vi "Generate SciScan specific XML params.vi"(8 "error in (no error)":errorcluster, 10 "DOM document IN":refnum<k20>, 11 "Non-Tree elements 2D array IN":string[][](array[string])) -> (0 "error out":errorcluster, 3 "Path-Value pairs Array":cluster{"XML Path":string, "XML Value":string}[](array[cluster]))   [LabVIEW 2012]
doc: "SciScan 1.2 160622"
uses:
  Custom Controls/file format type def.ctl
  Custom Controls/scan mode main settings tab.ctl
  GFG/GFGpathGet.vi
  GFG/GFG library.lvlib
  <resource>/objmgr/DOMUserDefRef.rc
  <vilib>/xml/NI_XML.lvlib
panel:
  out "node out":refnum<k20>
  in  "Channels 2 D Array IN":string[][](array[string])
  out "Array":string[](array[string])
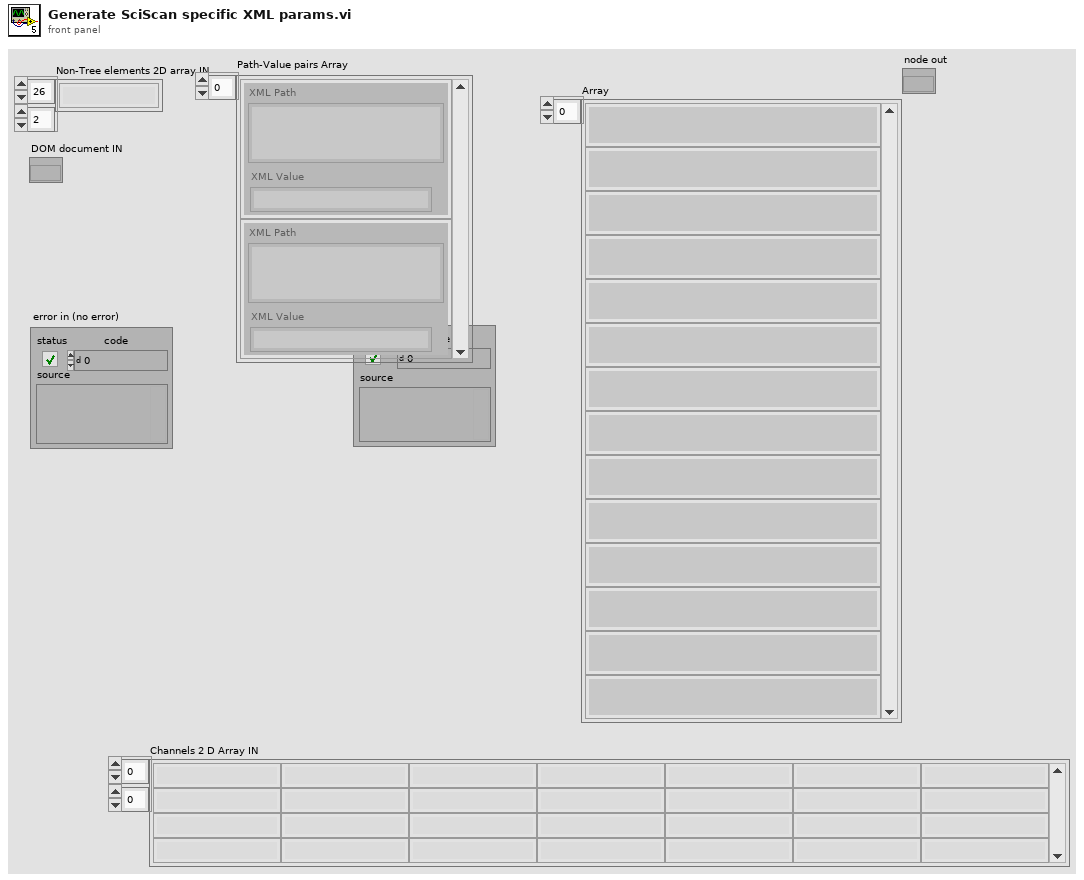
[diagram p1: front panel]
types:
  T1 = typedef "file format type def.ctl" = enum16{"16bit raw", "32bit raw", "16bit multi-tiff (interleave)", "16bit multi-tiff (separate)", "16bit multi-tiff (stacked)", "32bit multi-tiff (interleave)", "32bit multi-tiff (separate)", "32bit multi-tiff (stacked)", "16bit tiff series (interleave)", "16bit tiff series (separate)", "16bit tiff series (stacked)", "32bit tiff series (interleave)", "32bit tiff series (separate)", "32bit tiff series (stacked)"}
  T2 = typedef "scan mode main settings tab.ctl" = enum32{"2D frame", "2D line scan", "general settings", "Z Stack", "piezo"}
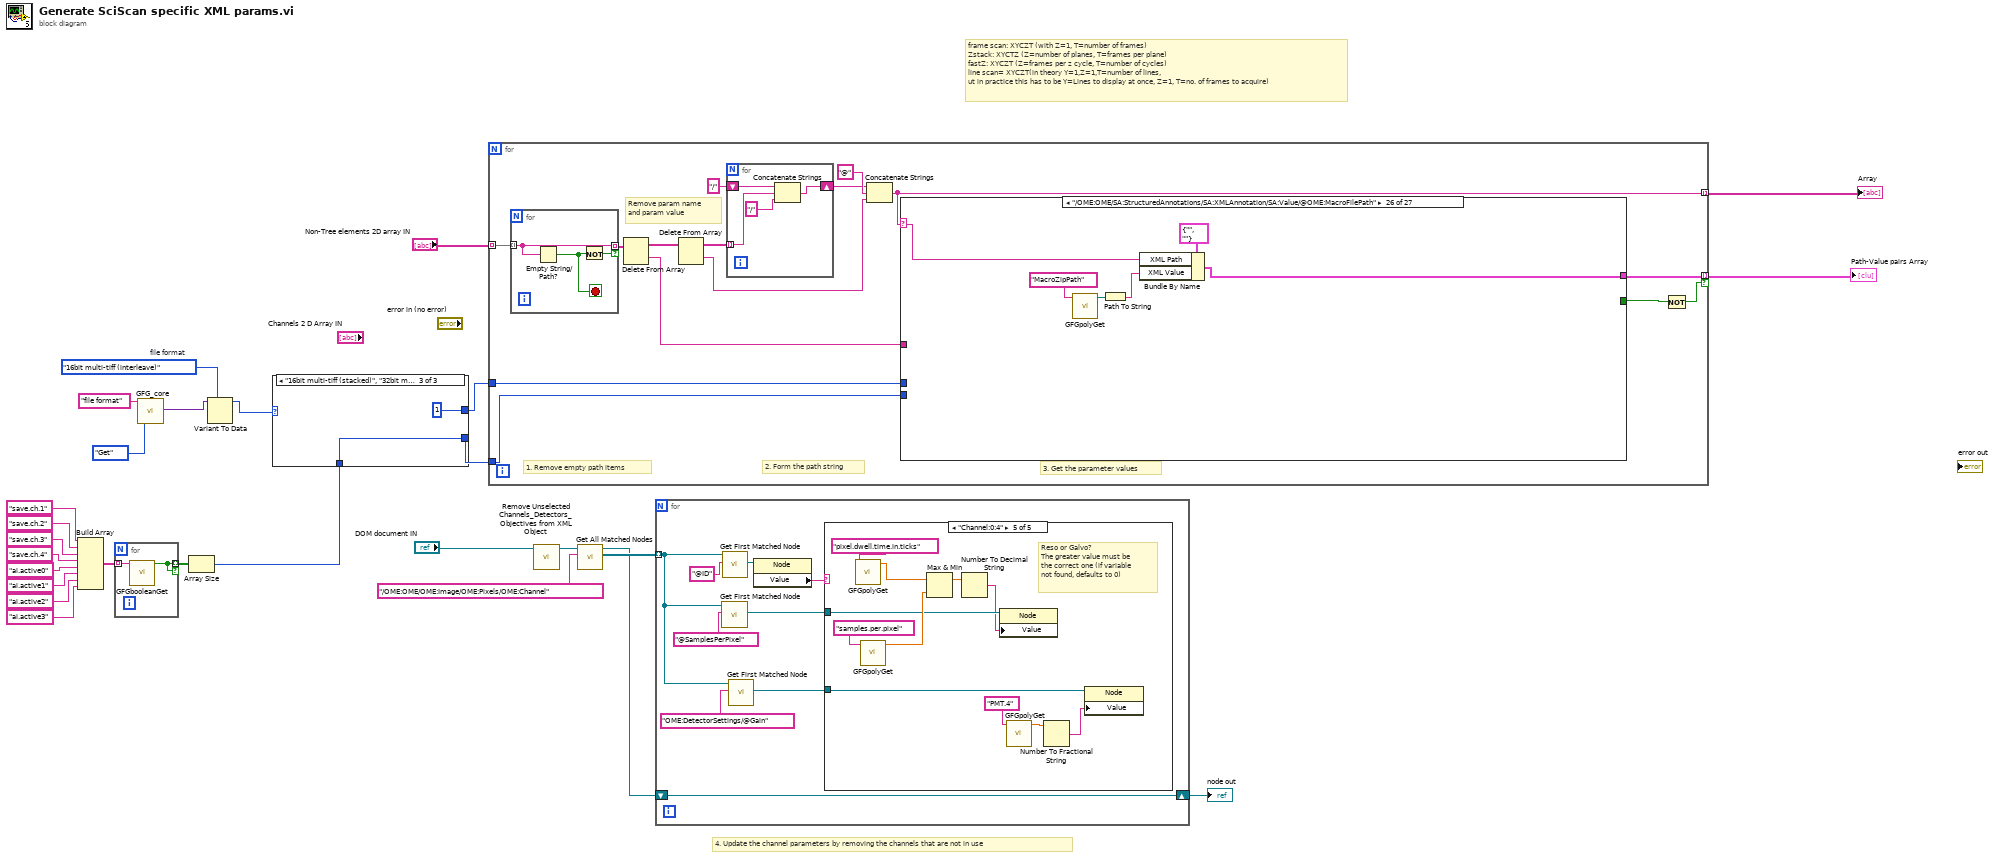
[diagram p0: block diagram]
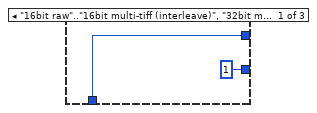
[diagram p2: hidden frame]
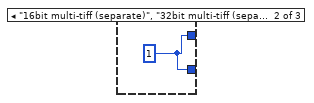
[diagram p3: hidden frame]
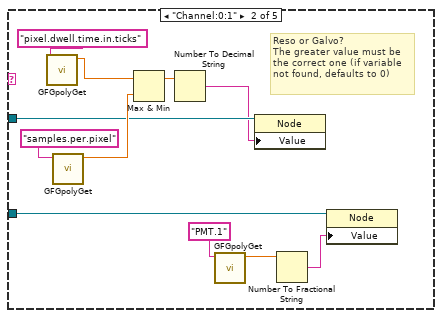
[diagram p5: hidden frame]
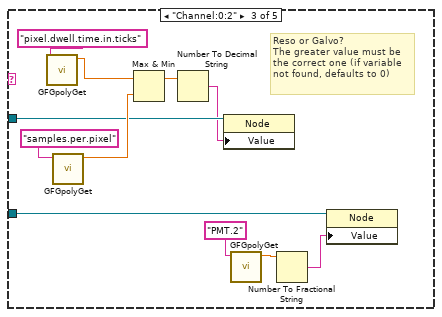
[diagram p6: hidden frame]
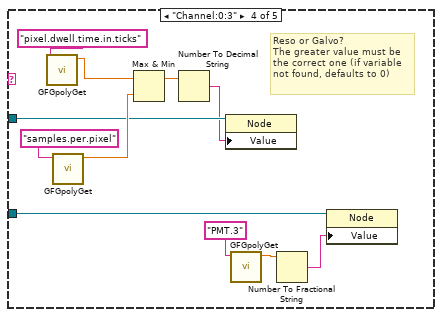
[diagram p7: hidden frame]
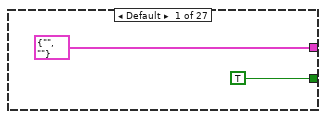
[diagram p8: hidden frame]
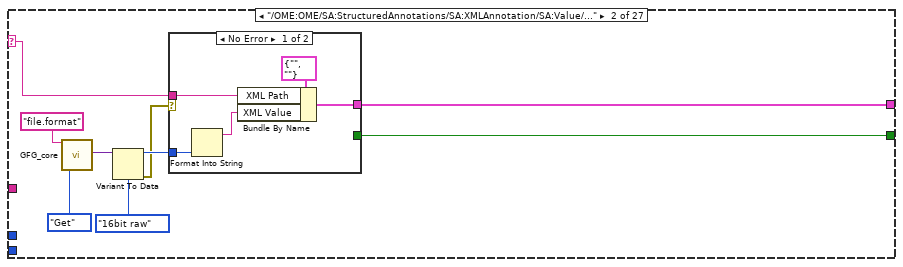
[diagram p9: hidden frame]
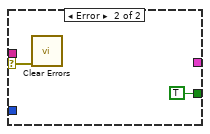
[diagram p10: hidden frame]
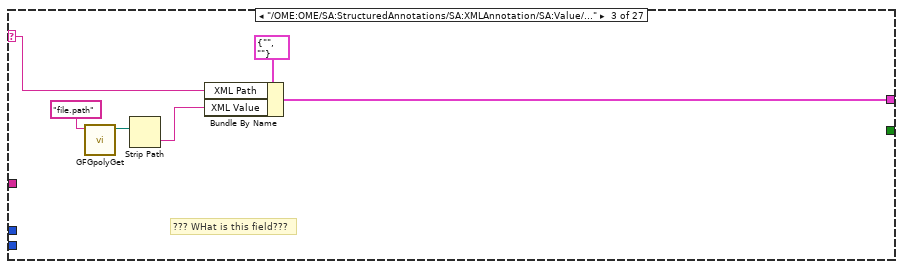
[diagram p11: hidden frame]
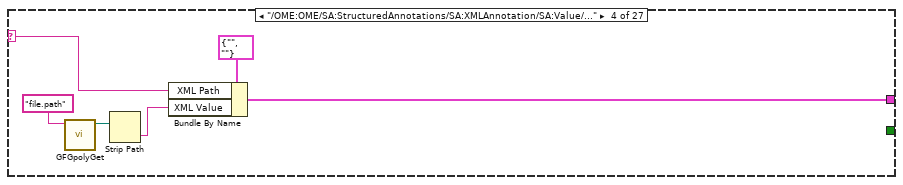
[diagram p12: hidden frame]
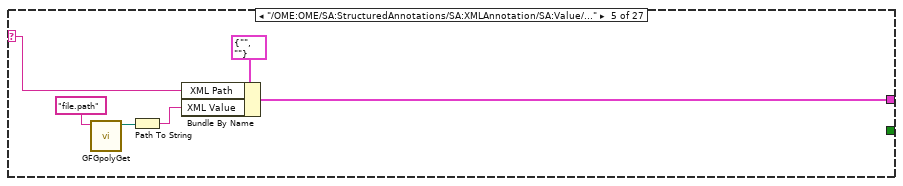
[diagram p13: hidden frame]
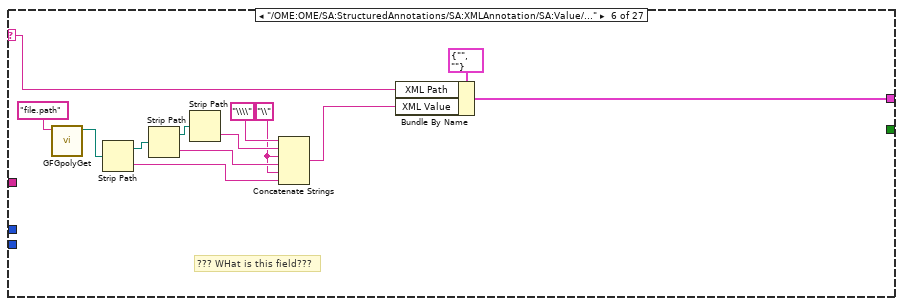
[diagram p14: hidden frame]
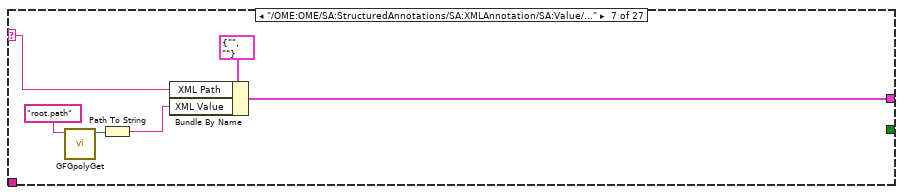
[diagram p15: hidden frame]
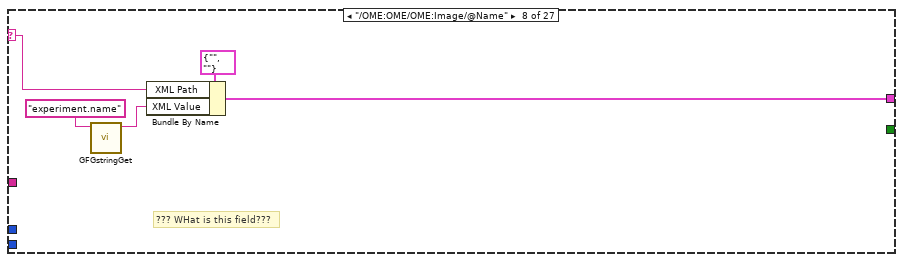
[diagram p16: hidden frame]
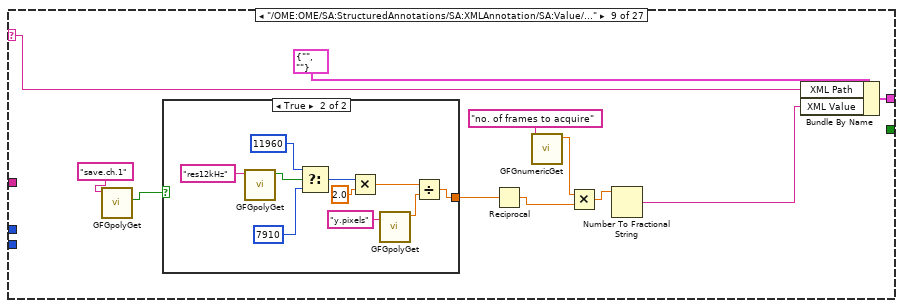
[diagram p17: hidden frame]
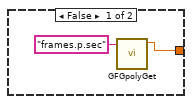
[diagram p18: hidden frame]
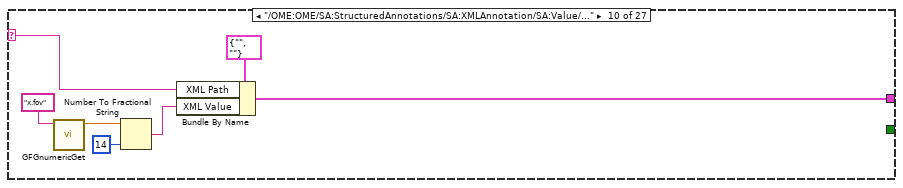
[diagram p19: hidden frame]
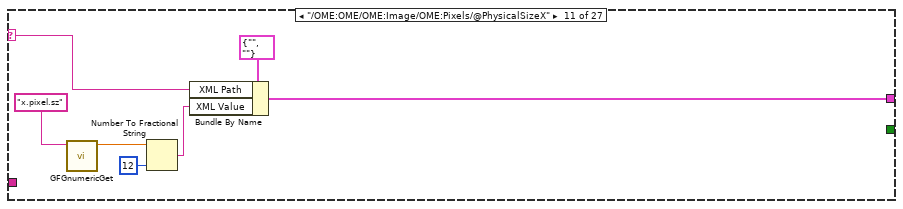
[diagram p20: hidden frame]
diagram:
  w16 = file_format_type_def."16bit multi-tiff (interleave)"  # file format
  # "frame scan: XYCZT (with Z=1, T=number of frames)\nZstack: XYCTZ (Z=number of planes, T=frames per plane)\nfastZ: XYCZT (Z=frames per z cycle, T=number of cycles)\nline scan= XYCZT(in theory Y=1,Z=1,T=number of lines, \nut in practice this has to be Y=Lines to display at once, Z=1, T=no. of frames to acquire)"
  # "4. Update the channel parameters by removing the channels that are not in use"
  n1 = Build Array("save.ch.1" ("Variable Name in"), "save.ch.2" ("Variable Name in"), "save.ch.3" ("Variable Name in"), "save.ch.4" ("Variable Name in"), "ai.active0" ("Variable Name in"), "ai.active1" ("Variable Name in"), "ai.active2" ("Variable Name in"), "ai.active3" ("Variable Name in")) -> (w14:string[])
  n2 = for {
    tunnel: w14 -> [w29] mode=indexing
    tunnel: [w28] -> w15 mode=indexing if=w28
    n3 = call "GFGbooleanGet.vi"("Variable Name in"=w29) -> ("Boolean Value OUT"=w28:bool)  [unwired: 9 in, 1 out]
  }
  n4 = call "GFG_core.vi"("Variable Name in"="file format", "Action"=enum16{"Init", "Set", "Get", "Clear"}."Get") -> ("Variant Out"=w17:variant)  [unwired: 11 in, 6 out]
  n5 = Array Size(array=w15) -> (size(s)=w4:i32)
  n6 = Variant To Data(type=w16, Variant=w17) -> (data=w5:T1)  [unwired: 1 in, 1 out]
  n7 = case shown="\"16bit multi-tiff (stacked)\", \"32bit multi-tiff (stacked)\", \"16bit tiff series (stacked)\", \"32bit tiff series (stacked)\"" w5 {
    tunnel: w4 -> [w30 _ w34]
    tunnel: [1 w32 w34] -> w3
    tunnel: [w30 w32 1] -> w2
    frame "16bit raw".."16bit multi-tiff (interleave)", "32bit multi-tiff (interleave)", "16bit tiff series (interleave)", "32bit tiff series (interleave)" {
    }
    frame "16bit multi-tiff (separate)", "32bit multi-tiff (separate)", "16bit tiff series (separate)", "32bit tiff series (separate)" {
      w32 = 1
    }
    frame "16bit multi-tiff (stacked)", "32bit multi-tiff (stacked)", "16bit tiff series (stacked)", "32bit tiff series (stacked)" {
    }
  }
  n8 = for {
    tunnel: "Non-Tree elements 2D array IN" -> [w43] mode=indexing
    tunnel: [w41] -> w27 mode=indexing
    tunnel: [w40] -> w26 mode=indexing if=w38
    tunnel: w3 -> [w36]
    tunnel: w2 -> [w35]
    # "3. Get the parameter values"
    # "2. Form the path string"
    # "1. Remove empty path items"
    # "Remove param name\nand param value"
    n9 = for {
      tunnel: w43 -> [w391] mode=indexing
      tunnel: [w391] -> w42 mode=indexing if=w390
      stop <- w392 stop-if-true
      n10 = Empty String/Path?(string/path=w391) -> (empty?=w392:bool)
      n11 = Not(x=w392) -> (.not. x?=w390:bool)
    }
    n12 = Delete From Array(array=w42) -> (deleted portion=w37:string, array with subset deleted=w47:string[])  [unwired: 2 in]
    n13 = Delete From Array(array=w47) -> (deleted portion=w44:string, array with subset deleted=w46:string[])  [unwired: 2 in]
    n14 = for {
      tunnel: w46 -> [w395] mode=indexing
      shift-right: [w393] -> w45
      shift-left: "/" ("string") -> [w396]
      n15 = Concatenate Strings(w396, w395, "/" ("string")) -> (w393:string)
    }
    n16 = Concatenate Strings(w45, "@" ("string"), w44) -> (w41:string)
    n17 = case shown="\"/OME:OME/SA:StructuredAnnotations/SA:XMLAnnotation/SA:Value/@OME:MacroFilePath\"" w41 {
      selector: w41 -> [_ w55 w70 w75 w81 w95 w100 w106 w119 w137 w146 w151 w159 w170 w180 w185 w210 w216 w223 w259 w265 w273 w306 w327 w349 w357 w367]
      tunnel: [cluster{"XML Path":string, "XML Value":string} {"XML Path"="", "XML Value"=""} ("Path-Value pairs") w56 w68 w74 w80 w94 w99 w105 w118 w138 w145 w150 w160 w163 w179 w186 w203 w218 w222 w258 w264 w272 w305 w326 w348 w356 w366] -> w40
      tunnel: [TRUE w52 _ _ _ _ _ _ _ _ _ _ _ _ _ w183 _ _ _ _ _ _ w307 w328 _ _ _] -> w39
      tunnel: w37 -> [_ _ _ _ _ _ _ _ _ _ _ _ _ _ _ _ _ _ _ _ _ _ _ _ _ _ _]
      tunnel: w36 -> [_ _ _ _ _ _ _ _ _ _ _ _ _ _ _ _ _ _ _ _ w266 _ _ _ _ _ _]
      tunnel: w35 -> [_ _ _ _ _ _ _ _ _ _ _ _ _ _ _ _ _ w219 _ _ _ _ _ _ _ _ _]
      frame Default {
      }
      frame "/OME:OME/SA:StructuredAnnotations/SA:XMLAnnotation/SA:Value/File/@Format" {
        n18 = call "GFG_core.vi"("Variable Name in"="file.format", "Action"=enum16{"Init", "Set", "Get", "Clear"}."Get") -> ("Variant Out"=w58:variant)  [unwired: 11 in, 6 out]
        n19 = Variant To Data(type=file_format_type_def."16bit raw" ("file format"), Variant=w58) -> (data=w57:T1, error out=w53:errorcluster)  [unwired: 1 in]
        n20 = case shown="No Error" w53 {
          selector: w53 -> [_ w67]
          tunnel: w57 -> [w65 _]
          tunnel: [w63 _] -> w56
          tunnel: w55 -> [w62 _]
          tunnel: [_ TRUE] -> w52
          frame No Error {
            n21 = Format Into String(w65) -> (resulting string=w61:string)  [unwired: 3 in, 1 out]
            n22 = Bundle By Name(cluster=cluster{"XML Path":string, "XML Value":string} {"XML Path"="", "XML Value"=""} ("Path-Value pairs"), "XML Path"=w62, "XML Value"=w61) -> (w63:cluster{"XML Path":string, "XML Value":string})
          }
          frame Error {
            n23 = call <vilib>:"Clear Errors.vi"("error in (no error)"=w67) -> ()  [unwired: 6 in, 1 out]
          }
        }
      }
      frame "/OME:OME/SA:StructuredAnnotations/SA:XMLAnnotation/SA:Value/File/@ID" {
        # "??? WHat is this field???"
        n24 = call-poly "GFGpolyGet.vi"("Variable Name in"="file.path" ("Tag in")) -> ("Path"=w72:path)  [unwired: 8 in, 2 out]
        n25 = Strip Path(path=w72) -> (name=w69:string)  [unwired: 1 out]
        n26 = Bundle By Name(cluster=cluster{"XML Path":string, "XML Value":string} {"XML Path"="", "XML Value"=""} ("Path-Value pairs"), "XML Path"=w70, "XML Value"=w69) -> (w68:cluster{"XML Path":string, "XML Value":string})
      }
      frame "/OME:OME/SA:StructuredAnnotations/SA:XMLAnnotation/SA:Value/File/@Name" {
        n27 = call-poly "GFGpolyGet.vi"("Variable Name in"="file.path" ("Tag in")) -> ("Path"=w78:path)  [unwired: 8 in, 2 out]
        n28 = Strip Path(path=w78) -> (name=w76:string)  [unwired: 1 out]
        n29 = Bundle By Name(cluster=cluster{"XML Path":string, "XML Value":string} {"XML Path"="", "XML Value"=""} ("Path-Value pairs"), "XML Path"=w75, "XML Value"=w76) -> (w74:cluster{"XML Path":string, "XML Value":string})
      }
      frame "/OME:OME/SA:StructuredAnnotations/SA:XMLAnnotation/SA:Value/File/@absPath" {
        n30 = call-poly "GFGpolyGet.vi"("Variable Name in"="file.path" ("Tag in")) -> ("Path"=w83:path)  [unwired: 8 in, 2 out]
        n31 = Path To String(path=w83) -> (string=w82:string)
        n32 = Bundle By Name(cluster=cluster{"XML Path":string, "XML Value":string} {"XML Path"="", "XML Value"=""} ("Path-Value pairs"), "XML Path"=w81, "XML Value"=w82) -> (w80:cluster{"XML Path":string, "XML Value":string})
      }
      frame "/OME:OME/SA:StructuredAnnotations/SA:XMLAnnotation/SA:Value/File/@relPath" {
        w86 = "\\" ("string")
        # "??? WHat is this field???"
        n33 = call-poly "GFGpolyGet.vi"("Variable Name in"="file.path" ("Tag in")) -> ("Path"=w97:path)  [unwired: 8 in, 2 out]
        n34 = Strip Path(path=w97) -> (stripped path=w93:path, name=w88:string)
        n35 = Strip Path(path=w93) -> (stripped path=w92:path, name=w89:string)
        n36 = Strip Path(path=w92) -> (name=w91:string)  [unwired: 1 out]
        n37 = Concatenate Strings("\\\\" ("string"), w91, w86, w89, w86, w88) -> (w87:string)
        n38 = Bundle By Name(cluster=cluster{"XML Path":string, "XML Value":string} {"XML Path"="", "XML Value"=""} ("Path-Value pairs"), "XML Path"=w95, "XML Value"=w87) -> (w94:cluster{"XML Path":string, "XML Value":string})
      }
      frame "/OME:OME/SA:StructuredAnnotations/SA:XMLAnnotation/SA:Value/File/@rootPath" {
        n39 = call-poly "GFGpolyGet.vi"("Variable Name in"="root.path" ("Tag in")) -> ("Path"=w102:path)  [unwired: 8 in, 2 out]
        n40 = Path To String(path=w102) -> (string=w101:string)
        n41 = Bundle By Name(cluster=cluster{"XML Path":string, "XML Value":string} {"XML Path"="", "XML Value"=""} ("Path-Value pairs"), "XML Path"=w100, "XML Value"=w101) -> (w99:cluster{"XML Path":string, "XML Value":string})
      }
      frame "/OME:OME/OME:Image/@Name" {
        # "??? WHat is this field???"
        n42 = call "GFGstringGet.vi"("Variable Name in"="experiment.name") -> ("String"=w107:string)  [unwired: 9 in, 1 out]
        n43 = Bundle By Name(cluster=cluster{"XML Path":string, "XML Value":string} {"XML Path"="", "XML Value"=""} ("Path-Value pairs"), "XML Path"=w106, "XML Value"=w107) -> (w105:cluster{"XML Path":string, "XML Value":string})
      }
      frame "/OME:OME/SA:StructuredAnnotations/SA:XMLAnnotation/SA:Value/ImagePhysicalDimensions/@PhysicalSizeT" {
        n44 = call-poly "GFGpolyGet.vi"("Variable Name in"="save.ch.1") -> ("Found/Replaced"=w110:bool)  [unwired: 9 in, 1 out]
        n45 = case shown="True" w110 {
          tunnel: [w122 w132] -> w117
          frame False {
            n46 = call-poly "GFGpolyGet.vi"("Variable Name in"="frames.p.sec") -> ("Numeric"=w122:dbl)  [unwired: 8 in, 2 out]
          }
          frame True {
            n47 = call-poly "GFGpolyGet.vi"("Variable Name in"="res12kHz") -> ("Boolean Value OUT"=w129:bool)  [unwired: 9 in, 1 out]
            n48 = Select(t=11960, s=w129, f=7910) -> (s? t:f=w130:i32)
            n49 = Multiply(x=w130, y=2.0) -> (x*y=w131:dbl)
            n50 = call-poly "GFGpolyGet.vi"("Variable Name in"="y.pixels") -> ("Numeric"=w124:dbl)  [unwired: 8 in, 2 out]
            n51 = Divide(x=w131, y=w124) -> (x/y=w132:dbl)
          }
        }
        n52 = Reciprocal(x=w117) -> (1/x=w114:dbl)
        n53 = call "GFGnumericGet.vi"("Variable Name in"="no. of frames to acquire") -> ("Numeric"=w113:dbl)  [unwired: 8 in, 2 out]
        n54 = Multiply(x=w113, y=w114) -> (x*y=w115:dbl)
        n55 = Number To Fractional String(number=w115) -> (F-format string=w116:string)  [unwired: 3 in]
        n56 = Bundle By Name(cluster=cluster{"XML Path":string, "XML Value":string} {"XML Path"="", "XML Value"=""} ("Path-Value pairs"), "XML Path"=w119, "XML Value"=w116) -> (w118:cluster{"XML Path":string, "XML Value":string})
      }
      frame "/OME:OME/SA:StructuredAnnotations/SA:XMLAnnotation/SA:Value/ImagePhysicalDimensions/@PhysicalSizeX" {
        n57 = call "GFGnumericGet.vi"("Variable Name in"="x.fov") -> ("Numeric"=w135:dbl)  [unwired: 8 in, 2 out]
        n58 = Number To Fractional String(number=w135, precision (6)=i16 14) -> (F-format string=w134:string)  [unwired: 2 in]
        n59 = Bundle By Name(cluster=cluster{"XML Path":string, "XML Value":string} {"XML Path"="", "XML Value"=""} ("Path-Value pairs"), "XML Path"=w137, "XML Value"=w134) -> (w138:cluster{"XML Path":string, "XML Value":string})
      }
      frame "/OME:OME/OME:Image/OME:Pixels/@PhysicalSizeX" {
        n60 = call "GFGnumericGet.vi"("Variable Name in"="x.pixel.sz") -> ("Numeric"=w143:dbl)  [unwired: 8 in, 2 out]
        n61 = Number To Fractional String(number=w143, precision (6)=i16 12) -> (F-format string=w144:string)  [unwired: 2 in]
        n62 = Bundle By Name(cluster=cluster{"XML Path":string, "XML Value":string} {"XML Path"="", "XML Value"=""} ("Path-Value pairs"), "XML Path"=w146, "XML Value"=w144) -> (w145:cluster{"XML Path":string, "XML Value":string})
      }
      frame "/OME:OME/SA:StructuredAnnotations/SA:XMLAnnotation/SA:Value/ImagePhysicalDimensions/@PhysicalSizeY" {
        n63 = call "GFGnumericGet.vi"("Variable Name in"="y.fov") -> ("Numeric"=w152:dbl)  [unwired: 8 in, 2 out]
        n64 = Number To Fractional String(number=w152, precision (6)=i16 14) -> (F-format string=w149:string)  [unwired: 2 in]
        n65 = Bundle By Name(cluster=cluster{"XML Path":string, "XML Value":string} {"XML Path"="", "XML Value"=""} ("Path-Value pairs"), "XML Path"=w151, "XML Value"=w149) -> (w150:cluster{"XML Path":string, "XML Value":string})
      }
      frame "/OME:OME/OME:Image/OME:Pixels/@PhysicalSizeY" {
        n66 = call "GFGnumericGet.vi"("Variable Name in"="y.pixel.sz") -> ("Numeric"=w157:dbl)  [unwired: 8 in, 2 out]
        n67 = Number To Fractional String(number=w157, precision (6)=i16 12) -> (F-format string=w158:string)  [unwired: 2 in]
        n68 = Bundle By Name(cluster=cluster{"XML Path":string, "XML Value":string} {"XML Path"="", "XML Value"=""} ("Path-Value pairs"), "XML Path"=w159, "XML Value"=w158) -> (w160:cluster{"XML Path":string, "XML Value":string})
      }
      frame "/OME:OME/SA:StructuredAnnotations/SA:XMLAnnotation/SA:Value/ImagePhysicalDimensions/@PhysicalSizeZ" {
        n69 = Build Array("piezo.active" ("Variable Name in"), "slow.z.stack" ("Variable Name in"), "start.z.stack" ("Variable Name in")) -> (w169:string[])
        n70 = for {
          tunnel: w169 -> [w172] mode=indexing
          tunnel: [w171] -> w165 mode=indexing
          n71 = call "GFGbooleanGet.vi"("Variable Name in"=w172) -> ("Boolean Value OUT"=w171:bool)  [unwired: 9 in, 1 out]
        }
        n72 = Or Array Elements(Boolean array=w165) -> (logical OR=w164:bool)
        n73 = case shown="True" w164 {
          tunnel: ["" w174] -> w162
          frame False {
          }
          frame True {
            n74 = call "GFGnumericGet.vi"("Variable Name in"="total.z.distance") -> ("Numeric"=w176:dbl)  [unwired: 8 in, 2 out]
            n75 = Number To Fractional String(number=w176) -> (F-format string=w174:string)  [unwired: 3 in]
          }
        }
        n76 = Bundle By Name(cluster=cluster{"XML Path":string, "XML Value":string} {"XML Path"="", "XML Value"=""} ("Path-Value pairs"), "XML Path"=w170, "XML Value"=w162) -> (w163:cluster{"XML Path":string, "XML Value":string})
      }
      frame "/OME:OME/OME:Image/@OME:AcquisitionDate" {
        # "Format to the style required in OME-XML"
        n77 = Get Date/Time In Seconds() -> (seconds since 1Jan1904=w181:timestamp)
        n78 = Format Date/Time String(seconds (now)=w181) -> ()  [unwired: 2 in, 1 out]
        n79 = Format Date/Time String(time format string (%c)="%Y-%m-%dT%H:%M:%S", seconds (now)=w181) -> (date/time string=w178:string)  [unwired: 1 in]
        n80 = Bundle By Name(cluster=cluster{"XML Path":string, "XML Value":string} {"XML Path"="", "XML Value"=""} ("Path-Value pairs"), "XML Path"=w180, "XML Value"=w178) -> (w179:cluster{"XML Path":string, "XML Value":string})
      }
      frame "/OME:OME/OME:Image/OME:Pixels/@BigEndian" {
        n81 = call "GFG_core.vi"("Variable Name in"="file.format", "Action"=enum16{"Init", "Set", "Get", "Clear"}."Get") -> ("Variant Out"=w190:variant)  [unwired: 11 in, 6 out]
        n82 = Variant To Data(type=file_format_type_def."16bit raw" ("file format"), Variant=w190) -> (data=w187:T1, error out=w184:errorcluster)  [unwired: 1 in]
        n83 = case shown="No Error" w184 {
          selector: w184 -> [_ w201]
          tunnel: w187 -> [w196 _]
          tunnel: [w194 _] -> w186
          tunnel: w185 -> [w193 _]
          tunnel: [_ TRUE] -> w183
          frame No Error {
            n84 = case shown="Default" w196 {
              tunnel: ["true" ("Variable Name in") "true" ("Variable Name in") "false" ("Variable Name in")] -> w192
              frame "16bit raw" {
              }
              frame "32bit raw" {
              }
              frame Default {
              }
            }
            n85 = Bundle By Name(cluster=cluster{"XML Path":string, "XML Value":string} {"XML Path"="", "XML Value"=""} ("Path-Value pairs"), "XML Path"=w193, "XML Value"=w192) -> (w194:cluster{"XML Path":string, "XML Value":string})
          }
          frame Error {
            n86 = call <vilib>:"Clear Errors.vi"("error in (no error)"=w201) -> ()  [unwired: 6 in, 1 out]
          }
        }
      }
      frame "/OME:OME/OME:Image/OME:Pixels/@DimensionOrder" {
        n87 = Build Array("slow.z.stack" ("Variable Name in"), "start.z.stack" ("Variable Name in")) -> (w209:string[])
        n88 = for {
          tunnel: w209 -> [w214] mode=indexing
          tunnel: [w213] -> w206 mode=indexing
          n89 = call "GFGbooleanGet.vi"("Variable Name in"=w214) -> ("Boolean Value OUT"=w213:bool)  [unwired: 9 in, 1 out]
        }
        n90 = Or Array Elements(Boolean array=w206) -> (logical OR=w205:bool)
        n91 = Select(t="XYCTZ" ("Variable Name in"), s=w205, f="XYCZT" ("Variable Name in")) -> (s? t:f=w204:string)
        n92 = Bundle By Name(cluster=cluster{"XML Path":string, "XML Value":string} {"XML Path"="", "XML Value"=""} ("Path-Value pairs"), "XML Path"=w210, "XML Value"=w204) -> (w203:cluster{"XML Path":string, "XML Value":string})
      }
      frame "/OME:OME/OME:Image/OME:Pixels/@SizeC" {
        # "Count for number of TRUE variables\n(for both Galvo and Reso)"
        n93 = Number To Decimal String(number=w219) -> (decimal integer string=w217:string)  [unwired: 1 in]
        n94 = Bundle By Name(cluster=cluster{"XML Path":string, "XML Value":string} {"XML Path"="", "XML Value"=""} ("Path-Value pairs"), "XML Path"=w216, "XML Value"=w217) -> (w218:cluster{"XML Path":string, "XML Value":string})
      }
      frame "/OME:OME/OME:Image/OME:Pixels/@SizeT" {
        # "frame scan: XYCZT (with Z=1, T=number of frames)\nZstack: XYCTZ (Z=number of planes, T=frames per plane)\nfastZ: XYCZT (Z=frames per z cycle, T=number of cycles)\nline scan= XYCZT(in theory Y=1,Z=1,T=number of lines, \nut in practice this has to be Y=Lines to display at once, Z=1, T=no. of frames to acquire)"
        # "Is it a line scan?"
        n95 = call "GFG_core.vi"("Variable Name in"="scan mode main settings") -> ("Found/Replaced"=w227:bool, "Variant Out"=w226:variant)  [unwired: 12 in, 5 out]
        n96 = case shown="True" w227 {
          tunnel: w226 -> [_ w254]
          tunnel: [_ w251] -> w225
          frame False {
          }
          frame True {
            n97 = Variant To Data(type=scan_mode_main_settings_tab."2D frame" ("scan mode main settings"), Variant=w254) -> (data=w252:T2)  [unwired: 1 in, 1 out]
            n98 = case shown="\"2D line scan\"" w252 {
              tunnel: [_ TRUE] -> w251
              frame Default {
              }
              frame "2D line scan" {
              }
            }
          }
        }
        n99 = case shown="True" w225 {
          tunnel: [w228 w248] -> w221
          frame False {
            n100 = call "GFGbooleanGet.vi"("Variable Name in"="piezo.active") -> ("Boolean Value OUT"=w229:bool)  [unwired: 9 in, 1 out]
            n101 = case shown="False" w229 {
              tunnel: [w236 w245] -> w228
              frame False {
                n102 = Build Array("slow.z.stack" ("Variable Name in"), "start.z.stack" ("Variable Name in")) -> (w235:string[])
                n103 = for {
                  tunnel: w235 -> [w238] mode=indexing
                  tunnel: [w237] -> w232 mode=indexing
                  n104 = call "GFGbooleanGet.vi"("Variable Name in"=w238) -> ("Boolean Value OUT"=w237:bool)  [unwired: 9 in, 1 out]
                }
                n105 = Or Array Elements(Boolean array=w232) -> (logical OR=w231:bool)
                n106 = case shown="False" w231 {
                  tunnel: [w239 w242] -> w236
                  frame False {
                    n107 = call "GFGnumericGet.vi"("Variable Name in"="no. of frames to acquire") -> ("Numeric"=w240:dbl)  [unwired: 8 in, 2 out]
                    n108 = Number To Decimal String(number=w240) -> (decimal integer string=w239:string)  [unwired: 1 in]
                  }
                  frame True {
                    n109 = call "GFGnumericGet.vi"("Variable Name in"="frames.per.plane") -> ("Numeric"=w243:dbl)  [unwired: 8 in, 2 out]
                    n110 = Number To Decimal String(number=w243) -> (decimal integer string=w242:string)  [unwired: 1 in]
                  }
                }
              }
              frame True {
                n111 = call "GFGnumericGet.vi"("Variable Name in"="no.of.cycles.to.scan") -> ("Numeric"=w246:dbl)  [unwired: 8 in, 2 out]
                n112 = Number To Decimal String(number=w246) -> (decimal integer string=w245:string)  [unwired: 1 in]
              }
            }
          }
          frame True {
            n113 = call "GFGnumericGet.vi"("Variable Name in"="no. of frames to acquire") -> ("Numeric"=w250:dbl)  [unwired: 8 in, 2 out]
            n114 = Number To Decimal String(number=w250) -> (decimal integer string=w248:string)  [unwired: 1 in]
          }
        }
        n115 = Bundle By Name(cluster=cluster{"XML Path":string, "XML Value":string} {"XML Path"="", "XML Value"=""} ("Path-Value pairs"), "XML Path"=w223, "XML Value"=w221) -> (w222:cluster{"XML Path":string, "XML Value":string})
      }
      frame "/OME:OME/OME:Image/OME:Pixels/@SizeX" {
        n116 = call "GFGnumericGet.vi"("Variable Name in"="nomin.x.pixels") -> ("Numeric"=w260:dbl)  [unwired: 8 in, 2 out]
        n117 = Number To Decimal String(number=w260) -> (decimal integer string=w257:string)  [unwired: 1 in]
        n118 = Bundle By Name(cluster=cluster{"XML Path":string, "XML Value":string} {"XML Path"="", "XML Value"=""} ("Path-Value pairs"), "XML Path"=w259, "XML Value"=w257) -> (w258:cluster{"XML Path":string, "XML Value":string})
      }
      frame "/OME:OME/OME:Image/OME:Pixels/@SizeY" {
        n119 = call "GFGnumericGet.vi"("Variable Name in"="y.pixels") -> ("Numeric"=w268:dbl)  [unwired: 8 in, 2 out]
        n120 = Multiply(x=w268, y=w266) -> (x*y=w267:dbl)
        n121 = Number To Decimal String(number=w267) -> (decimal integer string=w263:string)  [unwired: 1 in]
        n122 = Bundle By Name(cluster=cluster{"XML Path":string, "XML Value":string} {"XML Path"="", "XML Value"=""} ("Path-Value pairs"), "XML Path"=w265, "XML Value"=w263) -> (w264:cluster{"XML Path":string, "XML Value":string})
      }
      frame "/OME:OME/OME:Image/OME:Pixels/@SizeZ" {
        # "Is it a line scan?"
        n123 = call "GFG_core.vi"("Variable Name in"="scan mode main settings") -> ("Found/Replaced"=w277:bool, "Variant Out"=w276:variant)  [unwired: 12 in, 5 out]
        n124 = case shown="True" w277 {
          tunnel: w276 -> [_ w301]
          tunnel: [_ w298] -> w275
          frame False {
          }
          frame True {
            n125 = Variant To Data(type=scan_mode_main_settings_tab."2D frame" ("scan mode main settings"), Variant=w301) -> (data=w299:T2)  [unwired: 1 in, 1 out]
            n126 = case shown="\"2D line scan\"" w299 {
              tunnel: [_ TRUE] -> w298
              frame Default {
              }
              frame "2D line scan" {
              }
            }
          }
        }
        n127 = case shown="True" w275 {
          tunnel: [w278 "1"] -> w271
          frame False {
            n128 = call "GFGbooleanGet.vi"("Variable Name in"="piezo.active") -> ("Boolean Value OUT"=w279:bool)  [unwired: 9 in, 1 out]
            n129 = case shown="False" w279 {
              tunnel: [w286 w294] -> w278
              frame False {
                n130 = Build Array("slow.z.stack" ("Variable Name in"), "start.z.stack" ("Variable Name in")) -> (w285:string[])
                n131 = for {
                  tunnel: w285 -> [w288] mode=indexing
                  tunnel: [w287] -> w282 mode=indexing
                  n132 = call "GFGbooleanGet.vi"("Variable Name in"=w288) -> ("Boolean Value OUT"=w287:bool)  [unwired: 9 in, 1 out]
                }
                n133 = Or Array Elements(Boolean array=w282) -> (logical OR=w281:bool)
                n134 = case shown="True" w281 {
                  tunnel: [w290 w291] -> w286
                  frame False {
                    n135 = Number To Decimal String(number=1.0) -> (decimal integer string=w290:string)  [unwired: 1 in]
                  }
                  frame True {
                    n136 = call "GFGnumericGet.vi"("Variable Name in"="no of planes") -> ("Numeric"=w292:dbl)  [unwired: 8 in, 2 out]
                    n137 = Number To Decimal String(number=w292) -> (decimal integer string=w291:string)  [unwired: 1 in]
                  }
                }
              }
              frame True {
                n138 = call "GFGnumericGet.vi"("Variable Name in"="frames.per.z.cycle") -> ("Numeric"=w295:dbl)  [unwired: 8 in, 2 out]
                n139 = Number To Decimal String(number=w295) -> (decimal integer string=w294:string)  [unwired: 1 in]
              }
            }
          }
          frame True {
          }
        }
        n140 = Bundle By Name(cluster=cluster{"XML Path":string, "XML Value":string} {"XML Path"="", "XML Value"=""} ("Path-Value pairs"), "XML Path"=w273, "XML Value"=w271) -> (w272:cluster{"XML Path":string, "XML Value":string})
      }
      frame "/OME:OME/OME:Image/OME:Pixels/@Type" {
        n141 = call "GFG_core.vi"("Variable Name in"="file.format", "Action"=enum16{"Init", "Set", "Get", "Clear"}."Get") -> ("Variant Out"=w312:variant)  [unwired: 11 in, 6 out]
        n142 = Variant To Data(type=file_format_type_def."16bit raw" ("file format"), Variant=w312) -> (data=w309:T1, error out=w308:errorcluster)  [unwired: 1 in]
        n143 = case shown="No Error" w308 {
          selector: w308 -> [_ w323]
          tunnel: w309 -> [w319 _]
          tunnel: [w314 _] -> w304
          tunnel: [_ TRUE] -> w307
          frame No Error {
            # "If '16bit' found its a U16\n'32bit' implies float"
            n144 = Format Into String(w319) -> (resulting string=w318:string)  [unwired: 3 in, 1 out]
            n145 = Search/Split String(string=w318, search string/char (-)="16bit") -> (offset of match=w316:i32)  [unwired: 1 in, 2 out]
            n146 = Greater Or Equal To 0?(x=w316) -> (x >= 0?=w315:bool)
            n147 = case shown="False" w315 {
              tunnel: ["float" ("Variable Name in") "uint16" ("Variable Name in")] -> w314
              frame False {
              }
              frame True {
              }
            }
          }
          frame Error {
            n148 = call <vilib>:"Clear Errors.vi"("error in (no error)"=w323) -> ()  [unwired: 6 in, 1 out]
          }
        }
        n149 = Bundle By Name(cluster=cluster{"XML Path":string, "XML Value":string} {"XML Path"="", "XML Value"=""} ("Path-Value pairs"), "XML Path"=w306, "XML Value"=w304) -> (w305:cluster{"XML Path":string, "XML Value":string})
      }
      frame "/OME:OME/OME:Image/OME:Pixels/@SignificantBits" {
        n150 = call "GFG_core.vi"("Variable Name in"="file.format", "Action"=enum16{"Init", "Set", "Get", "Clear"}."Get") -> ("Variant Out"=w333:variant)  [unwired: 11 in, 6 out]
        n151 = Variant To Data(type=file_format_type_def."16bit raw" ("file format"), Variant=w333) -> (data=w330:T1, error out=w329:errorcluster)  [unwired: 1 in]
        n152 = case shown="No Error" w329 {
          selector: w329 -> [_ w344]
          tunnel: w330 -> [w340 _]
          tunnel: [w335 _] -> w325
          tunnel: [_ TRUE] -> w328
          frame No Error {
            # "If '16bit' found its a U16\n'32bit' implies float"
            n153 = Format Into String(w340) -> (resulting string=w339:string)  [unwired: 3 in, 1 out]
            n154 = Search/Split String(string=w339, search string/char (-)="16bit") -> (offset of match=w337:i32)  [unwired: 1 in, 2 out]
            n155 = Greater Or Equal To 0?(x=w337) -> (x >= 0?=w336:bool)
            n156 = case shown="False" w336 {
              tunnel: ["32" ("Variable Name in") "16" ("Variable Name in")] -> w335
              frame False {
              }
              frame True {
              }
            }
          }
          frame Error {
            n157 = call <vilib>:"Clear Errors.vi"("error in (no error)"=w344) -> ()  [unwired: 6 in, 1 out]
          }
        }
        n158 = Bundle By Name(cluster=cluster{"XML Path":string, "XML Value":string} {"XML Path"="", "XML Value"=""} ("Path-Value pairs"), "XML Path"=w327, "XML Value"=w325) -> (w326:cluster{"XML Path":string, "XML Value":string})
      }
      frame "/OME:OME/SA:StructuredAnnotations/SA:XMLAnnotation/SA:Value/@PixelDwellTime" {
        n159 = call "GFGnumericGet.vi"("Variable Name in"="pixel.dwell.time.in.sec") -> ("Numeric"=w350:dbl)  [unwired: 8 in, 2 out]
        n160 = Number To Fractional String(number=w350, precision (6)=i16 12) -> (F-format string=w347:string)  [unwired: 2 in]
        n161 = Bundle By Name(cluster=cluster{"XML Path":string, "XML Value":string} {"XML Path"="", "XML Value"=""} ("Path-Value pairs"), "XML Path"=w349, "XML Value"=w347) -> (w348:cluster{"XML Path":string, "XML Value":string})
      }
      frame "/OME:OME/SA:StructuredAnnotations/SA:XMLAnnotation/SA:Value/@OME:MacroFilePath" {
        n162 = call-poly "GFGpolyGet.vi"("Variable Name in"="MacroZipPath") -> ("Path"=w353:path)  [unwired: 8 in, 2 out]
        n163 = Path To String(path=w353) -> (string=w352:string)
        n164 = Bundle By Name(cluster=cluster{"XML Path":string, "XML Value":string} {"XML Path"="", "XML Value"=""} ("Path-Value pairs"), "XML Path"=w357, "XML Value"=w352) -> (w356:cluster{"XML Path":string, "XML Value":string})
      }
      frame "/OME:OME/SA:StructuredAnnotations/SA:XMLAnnotation/SA:Value/@LaserPower" {
        n165 = Build Array("piezo.active" ("Variable Name in"), "slow.z.stack" ("Variable Name in"), "start.z.stack" ("Variable Name in")) -> (w363:string[])
        n166 = for {
          tunnel: w363 -> [w369] mode=indexing
          tunnel: [w368] -> w359 mode=indexing
          n167 = call "GFGbooleanGet.vi"("Variable Name in"=w369) -> ("Boolean Value OUT"=w368:bool)  [unwired: 9 in, 1 out]
        }
        n168 = Or Array Elements(Boolean array=w359) -> (logical OR=w358:bool)
        n169 = case shown="True" w358 {
          tunnel: [w370 w376] -> w365
          frame False {
            n170 = call "GFGnumericGet.vi"("Variable Name in"="Laser.Power") -> ("Numeric"=w371:dbl)  [unwired: 8 in, 2 out]
            n171 = Number To Fractional String(number=w371) -> (F-format string=w370:string)  [unwired: 3 in]
          }
          frame True {
            w389 = 3 ("disabled index (col)")
            # "Last row index"
            n172 = call "GFG_core.vi"("Variable Name in"="pos  pockels cell PMT Data") -> ("Variant Out"=w383:variant)  [unwired: 12 in, 6 out]
            n173 = Variant To Data(type=dbl[][] [] ("Interpolated Data"), Variant=w383) -> (data=w382:dbl[][], error out=w373:errorcluster)  [unwired: 1 in]
            n174 = call <vilib>:"Clear Errors.vi"("error in (no error)"=w373) -> ()  [unwired: 6 in, 1 out]
            n175 = Array Size(array=w382) -> (size(s)=w385:i32[])
            n176 = Index Array(array=w385, index=0) -> (element=w386:i32)
            n177 = Decrement(x=w386) -> (x-1=w375:i32)
            n178 = Index Array(array=w382, index (row)=0, index (col)=w389) -> (element=w381:dbl)
            n179 = Index Array(array=w382, index (row)=w375, index (col)=w389) -> (element=w380:dbl)
            n180 = Number To Fractional String(number=w381) -> (F-format string=w378:string)  [unwired: 3 in]
            n181 = Number To Fractional String(number=w380) -> (F-format string=w379:string)  [unwired: 3 in]
            n182 = Concatenate Strings(w378, " - " ("string"), w379) -> (w376:string)
          }
        }
        n183 = Bundle By Name(cluster=cluster{"XML Path":string, "XML Value":string} {"XML Path"="", "XML Value"=""} ("Path-Value pairs"), "XML Path"=w367, "XML Value"=w365) -> (w366:cluster{"XML Path":string, "XML Value":string})
      }
    }
    n184 = Not(x=w39) -> (.not. x?=w38:bool)
  }
  "Path-Value pairs Array" <- w26
  "Array" <- w27
  n185 = call "Remove Unselected Channels_Detectors_Objectives from XML Object.vi"("Document Refnum IN"="DOM document IN") -> ("Document Refnum Out"=w24:refnum<k20>)  [unwired: 9 in, 1 out]
  n186 = call <vilib>:"Get All Matched Nodes.vi"("XPath expression"="/OME:OME/OME:Image/OME:Pixels/OME:Channel", "node in"=w24) -> ("node result array"=w22:refnum<k20>[], "node out"=w21:refnum<k20>)  [unwired: 7 in, 1 out]
  n187 = for {
    tunnel: w22 -> [w398] mode=indexing
    shift-right: [w400] -> w20
    shift-left: w21 -> [w400]
    n188 = call <vilib>:"Get First Matched Node.vi"("XPath expression"="@SamplesPerPixel", "node in"=w398) -> ("node result"=w397:refnum<k20>)  [unwired: 7 in, 2 out]
    n189 = call <vilib>:"Get First Matched Node.vi"("XPath expression"="@ID", "node in"=w398) -> ("node result"=w404:refnum<k20>)  [unwired: 7 in, 2 out]
    n190 = call <vilib>:"Get First Matched Node.vi"("XPath expression"="OME:DetectorSettings/@Gain", "node in"=w398) -> ("node result"=w401:refnum<k20>)  [unwired: 7 in, 2 out]
    n191 = property class="Node"(reference=w404) -> ("Value"=w403:string)  [unwired: 1 in, 2 out]
    n192 = case shown="\"Channel:0:4\"" w403 {
      tunnel: w401 -> [_ w408 w419 w430 w441]
      tunnel: w397 -> [_ w407 w418 w429 w440]
      frame Default {
      }
      frame "Channel:0:1" {
        # "Reso or Galvo?\nThe greater value must be \nthe correct one (if variable\nnot found, defaults to 0)"
        n193 = call-poly "GFGpolyGet.vi"("Variable Name in"="pixel.dwell.time.in.ticks") -> ("Numeric"=w414:dbl)  [unwired: 8 in, 2 out]
        n194 = call-poly "GFGpolyGet.vi"("Variable Name in"="samples.per.pixel") -> ("Numeric"=w413:dbl)  [unwired: 8 in, 2 out]
        n195 = Max & Min(x=w414, y=w413) -> (max(x,y)=w412:dbl)  [unwired: 1 out]
        n196 = Number To Decimal String(number=w412) -> (decimal integer string=w406:string)  [unwired: 1 in]
        n197 = call-poly "GFGpolyGet.vi"("Variable Name in"="PMT.1") -> ("Numeric"=w410:dbl)  [unwired: 8 in, 2 out]
        n198 = property class="Node"(reference=w407, "Value"=w406) -> ()  [unwired: 1 in, 2 out]
        n199 = Number To Fractional String(number=w410) -> (F-format string=w409:string)  [unwired: 3 in]
        n200 = property class="Node"(reference=w408, "Value"=w409) -> ()  [unwired: 1 in, 2 out]
      }
      frame "Channel:0:2" {
        # "Reso or Galvo?\nThe greater value must be \nthe correct one (if variable\nnot found, defaults to 0)"
        n201 = call-poly "GFGpolyGet.vi"("Variable Name in"="pixel.dwell.time.in.ticks") -> ("Numeric"=w425:dbl)  [unwired: 8 in, 2 out]
        n202 = call-poly "GFGpolyGet.vi"("Variable Name in"="samples.per.pixel") -> ("Numeric"=w424:dbl)  [unwired: 8 in, 2 out]
        n203 = Max & Min(x=w425, y=w424) -> (max(x,y)=w423:dbl)  [unwired: 1 out]
        n204 = Number To Decimal String(number=w423) -> (decimal integer string=w417:string)  [unwired: 1 in]
        n205 = property class="Node"(reference=w418, "Value"=w417) -> ()  [unwired: 1 in, 2 out]
        n206 = call-poly "GFGpolyGet.vi"("Variable Name in"="PMT.2") -> ("Numeric"=w421:dbl)  [unwired: 8 in, 2 out]
        n207 = Number To Fractional String(number=w421) -> (F-format string=w420:string)  [unwired: 3 in]
        n208 = property class="Node"(reference=w419, "Value"=w420) -> ()  [unwired: 1 in, 2 out]
      }
      frame "Channel:0:3" {
        # "Reso or Galvo?\nThe greater value must be \nthe correct one (if variable\nnot found, defaults to 0)"
        n209 = call-poly "GFGpolyGet.vi"("Variable Name in"="pixel.dwell.time.in.ticks") -> ("Numeric"=w436:dbl)  [unwired: 8 in, 2 out]
        n210 = call-poly "GFGpolyGet.vi"("Variable Name in"="samples.per.pixel") -> ("Numeric"=w435:dbl)  [unwired: 8 in, 2 out]
        n211 = Max & Min(x=w436, y=w435) -> (max(x,y)=w434:dbl)  [unwired: 1 out]
        n212 = Number To Decimal String(number=w434) -> (decimal integer string=w428:string)  [unwired: 1 in]
        n213 = property class="Node"(reference=w429, "Value"=w428) -> ()  [unwired: 1 in, 2 out]
        n214 = call-poly "GFGpolyGet.vi"("Variable Name in"="PMT.3") -> ("Numeric"=w432:dbl)  [unwired: 8 in, 2 out]
        n215 = Number To Fractional String(number=w432) -> (F-format string=w431:string)  [unwired: 3 in]
        n216 = property class="Node"(reference=w430, "Value"=w431) -> ()  [unwired: 1 in, 2 out]
      }
      frame "Channel:0:4" {
        # "Reso or Galvo?\nThe greater value must be \nthe correct one (if variable\nnot found, defaults to 0)"
        n217 = call-poly "GFGpolyGet.vi"("Variable Name in"="pixel.dwell.time.in.ticks") -> ("Numeric"=w447:dbl)  [unwired: 8 in, 2 out]
        n218 = call-poly "GFGpolyGet.vi"("Variable Name in"="samples.per.pixel") -> ("Numeric"=w446:dbl)  [unwired: 8 in, 2 out]
        n219 = Max & Min(x=w447, y=w446) -> (max(x,y)=w445:dbl)  [unwired: 1 out]
        n220 = Number To Decimal String(number=w445) -> (decimal integer string=w439:string)  [unwired: 1 in]
        n221 = property class="Node"(reference=w440, "Value"=w439) -> ()  [unwired: 1 in, 2 out]
        n222 = call-poly "GFGpolyGet.vi"("Variable Name in"="PMT.4") -> ("Numeric"=w443:dbl)  [unwired: 8 in, 2 out]
        n223 = Number To Fractional String(number=w443) -> (F-format string=w442:string)  [unwired: 3 in]
        n224 = property class="Node"(reference=w441, "Value"=w442) -> ()  [unwired: 1 in, 2 out]
      }
    }
  }
  "node out" <- w20
